vi "RTC时钟实验.vi"() -> ()   [LabVIEW 2011]
uses:
  <vilib>/STM32_DriverVI_Interface_F4/RTC/RTC_ClK_Source_F4xx.ctl
panel:
  out "Hour":u8=8
  out "Minute":u8=8
  out "Second":u8=8
  out "AM/PM":enum8{"AM/24H", "PM"}(ring)
  out "Week":T1(ring)
  out "Day":u8=25
  out "Month":u8=7
  out "Year":u16=2013
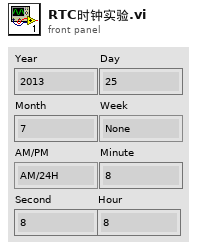
[diagram p1: front panel]
types:
  T1 = enum8{"None", "Monday", "Tuesday", "Wednesday", "Thursday", "Friday", "Saturday", "Sunday"}
  T2 = typedef "RTC_ClK_Source_F4xx.ctl" = enum8{"外部:32.768KHz", "内部:LSI: 40KHz"}
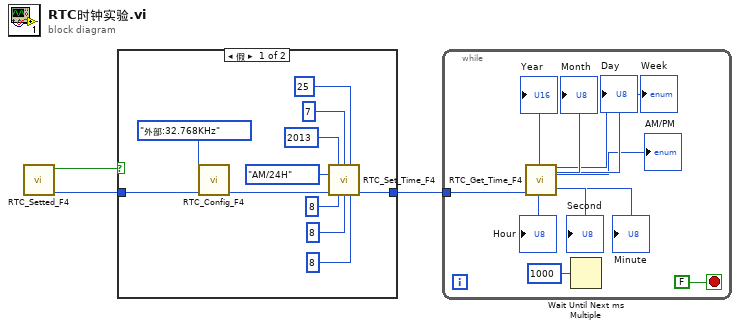
[diagram p0: block diagram]
diagram:
  n1 = call <vilib>:"RTC_Setted_F4.vi"() -> ("err_out"=w2:u8, "RTC是否已经设置过？"=w3:bool)  [unwired: 10 in]
  n2 = case shown="假" w3 {
    tunnel: w2 -> [w14 _]
    tunnel: [w5 _] -> w1
    frame False {
      n3 = call <vilib>:"RTC_Config_F4.vi"("err_in"=w14, "RTC_CLK_Source_F4"=RTC_ClK_Source_F4xx."外部:32.768KHz") -> ("err_out"=w13:u8)  [unwired: 8 in, 1 out]
      n4 = call <vilib>:"RTC_Set_Time_F4.vi"("Year（2000~2099）"=u16 2013, "Month"=u8 7, "Day"=u8 25, "AM/PM"=enum8{"AM/24H", "PM"}."AM/24H", "err_in"=w13, "Hour"=u8 8, "Minute"=u8 8, "Second"=u8 8) -> ("err_out"=w5:u8)  [unwired: 7 in]
    }
    frame True {
    }
  }
  n5 = while {
    tunnel: w1 -> [w25]
    stop <- FALSE stop-if-true
    n6 = call <vilib>:"RTC_Get_Time_F4.vi"("err_in"=w25) -> ("Year"=→"Year":u16, "Month"=→"Month":u8, "Day"=→"Day":u8, "Week"=→"Week":T1, "AM/PM"=→"AM/PM":enum8{"AM/24H", "PM"}, "Hour"=→"Hour":u8, "Minute"=→"Minute":u8, "Second"=→"Second":u8)  [unwired: 6 in, 1 out]
    n7 = Wait Until Next ms Multiple(millisecond multiple=u32 1000 ("毫秒倍数")) -> ()  [unwired: 1 out]
  }
